vi "Parse ID Token elements.vi"(8 "error in (no error)":errorcluster, 11 "ID Token":string) -> (0 "error out":errorcluster, 1 "signature":string, 2 "payload":string, 3 "header":string)   [LabVIEW 2017, in "JSONWebToken.lvclass"]
uses:
  JSONWebToken.lvclass
  <vilib>/Utility/error.llb/Error Cluster From Error Code.vi
  <vilib>/ErrorRing/Error Ring.xnode
  <vilib>/LabVIEW Open Source Project/OpenSerializer.Base64/Serializer.Base64.lvclass
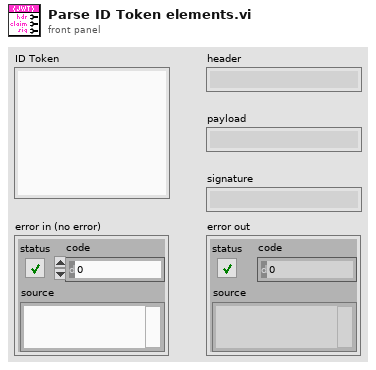
[diagram p1: front panel]
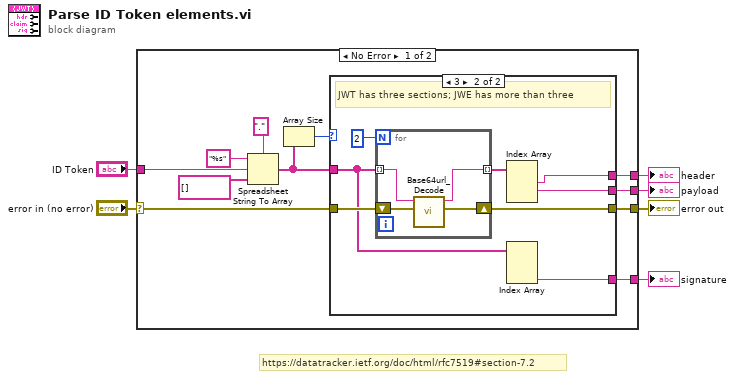
[diagram p0: block diagram]
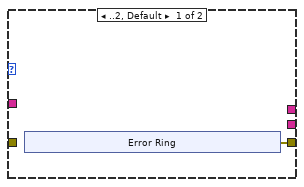
[diagram p2: hidden frame]
diagram:
  # "https://datatracker.ietf.org/doc/html/rfc7519#section-7.2"
  n1 = case shown="No Error" "error in (no error)" {
    selector: "error in (no error)" -> [w12 w35]
    tunnel: "ID Token" -> [w16 _]
    tunnel: [w15 _] -> w5
    tunnel: [w14 _] -> w4
    tunnel: [w11 _] -> w3
    tunnel: [w13 w35] -> w2
    frame No Error {
      n2 = Spreadsheet String To Array(delimiter (Tab)="." ("delimiter"), format string="%s", spreadsheet string=w16, array type (2D Dbl)=string[] []) -> (array=w10:string[])
      n3 = Array Size(array=w10) -> (size(s)=w9:i32)
      n4 = case shown="3" w9 {
        tunnel: [_ w28] -> w15
        tunnel: [_ w27] -> w14
        tunnel: [w18 w26] -> w13
        tunnel: w12 -> [_ w25]
        tunnel: w10 -> [_ w24]
        tunnel: [_ w23] -> w11
        frame ..2, Default {
          n5 = xnode "Error Ring"() -> ("error out"=w18:errorcluster)
        }
        frame 3 {
          # "JWT has three sections; JWE has more than three"
          n6 = for {
            N: 2 -> [_]
            tunnel: w24 -> [w31] mode=indexing
            tunnel: [w32] -> w29 mode=indexing
            shift-right: [w34] -> w26
            shift-left: w25 -> [w33]
            n7 = call <vilib>:"Base64url_Decode.vi"("error in (no error)"=w33, "Base64 URL String"=w31) -> ("error out"=w34:errorcluster, "Decoded String"=w32:string)  [unwired: 8 in]
          }
          n8 = Index Array(array=w29) -> (element #1=w28:string, element #2=w27:string)  [unwired: 3 in, 1 out]
          n9 = Index Array(array=w24) -> (element #3=w23:string)  [unwired: 3 in, 2 out]
        }
      }
    }
    frame Error {
    }
  }
  "payload" <- w4
  "error out" <- w2
  "header" <- w5
  "signature" <- w3
